vi "Joystick Home Fix.vi"(11 "Joystick Input":dbl) -> (3 "Power % Output":dbl)   [LabVIEW 2016]
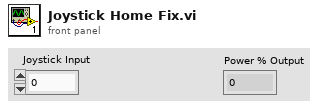
[diagram p1: front panel]
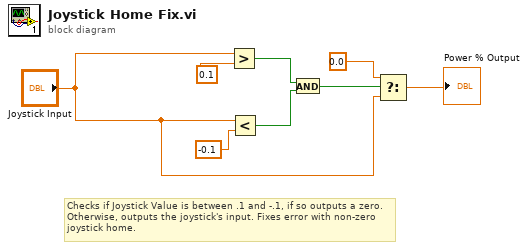
[diagram p0: block diagram]
diagram:
  # "Checks if Joystick Value is between .1 and -.1, if so outputs a zero.\nOtherwise, outputs the joystick's input. Fixes error with non-zero\njoystick home."
  n1 = Greater?(x="Joystick Input", y=0.1) -> (0:w8:bool)
  n2 = Less?(x="Joystick Input", y=-0.1) -> (x < y?=w7:bool)
  n3 = And(x=w8, y=w7) -> (x .and. y?=w5:bool)
  n4 = Select(t=0.0, s=w5, f="Joystick Input") -> (s? t:f=→"Power % Output":dbl)
